vi "UART Benchmark.vi"() -> ()   [LabVIEW 2011]
uses:
  Private/Device/Device.lvlib
  Private/Type Defs/Interface.ctl
  LVH-LINX.lvlib
  <vilib>/ptbypt/NI_PtbyPt.lvlib
panel:
  in  "Data":string
  out "Device Name":string
  in  "Stop Button":bool
  out "Loop Rate":dbl(graph)
  out "Loop Time (ms)":i32
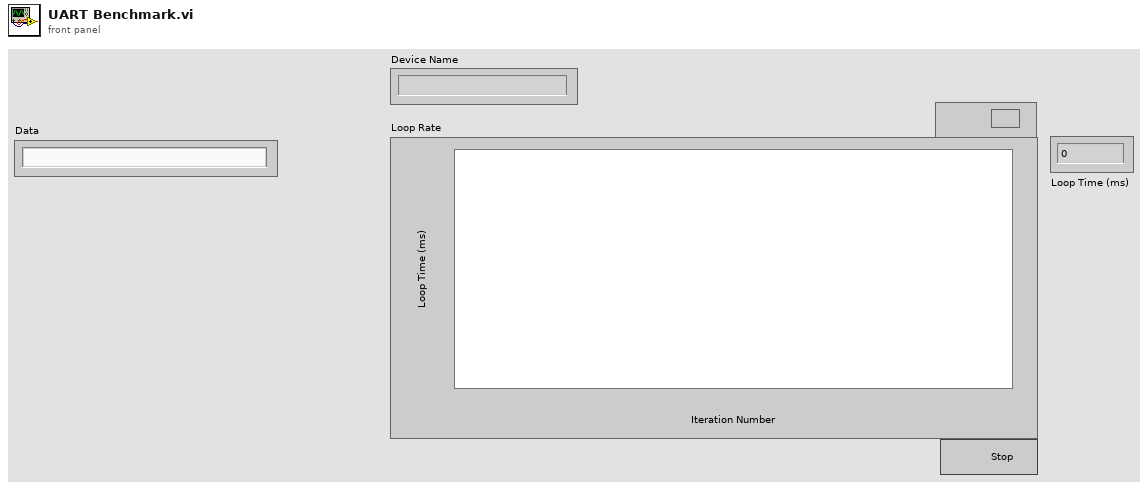
[diagram p1: front panel]
types:
  T1 = typedef "LVH-LINX.lvlib/Interface.ctl" = enum16{"Serial", "TCP"}
  T2 = typedef "LVH-LINX.lvlib/Device.lvlib/LINX Device Config.ctl" = cluster{"Interface":T1, "COM Port":refnum<visa-resource-name>, "TCP Configuration":T3, "Device Family":u8, "Device ID":u8, "Device Name":string, "TCP Ref":refnum<k5>, "Channels":T4}
  T3 = typedef "LVH-LINX.lvlib/Device.lvlib/TCP Config.ctl" = cluster{"IP Address":string, "Port":u16}
  T4 = typedef "LVH-LINX.lvlib/Channels.ctl" = cluster{"DI Channels":u8[], "DO Channels":u8[], "AI":u8[], "AO":u8[], "PWM":u8[], "QE":u8[], "UART":u8[], "I2C 2":u8[], "SPI":u8[], "CAN":u8[], "AI Ref (V)":dbl, "AO Resolution (Bits)":u8, "AO Ref (V)":dbl}
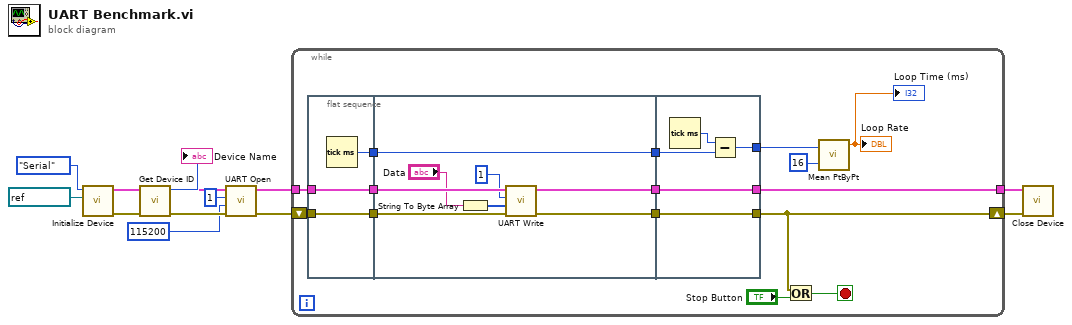
[diagram p0: block diagram]
diagram:
  n1 = call "Initialize Device.vi"("COM Port"=refnum<visa-resource-name> "COM5", "Interface"=Interface."Serial") -> ("Error Out"=w9:errorcluster, "LINX Device Config"=w10:T2)  [unwired: 8 in]
  n2 = call "Get Device ID.vi"("Error In"=w9, "LINX Device Config"=w10) -> ("Error Out"=w7:errorcluster, "Device Family"=→"Device Name":u8, "LINX Device Config"=w6:T2)  [unwired: 6 in, 1 out]
  n3 = call "UART Open.vi"("Error In"=w7, "Baud Rate (9600)"=u32 115200, "UART Channel"=u8 1, "LINX Device Config"=w6) -> ("Error Out"=w3:errorcluster, "LINX Device Config"=w2:T2)  [unwired: 6 in]
  n4 = while {
    shift-right: [w14] -> w11
    shift-left: w3 -> [w21]
    tunnel: w2 -> [w17]
    tunnel: [w16] -> w1
    stop <- w28 stop-if-true
    n5 = flat-sequence {
      tunnel: [w31] -> w26
      tunnel: w21 -> [w30]
      tunnel: [w30] -> w20
      tunnel: [w29] -> w18
      tunnel: w17 -> [w29]
      tunnel: w26 -> [w39]
      tunnel: [w39] -> w25
      tunnel: w20 -> [w38]
      tunnel: [w37] -> w19
      tunnel: w18 -> [w36]
      tunnel: [w35] -> w15
      tunnel: w25 -> [w43]
      tunnel: [w42] -> w24
      tunnel: [w41] -> w14
      tunnel: w19 -> [w41]
      tunnel: [w40] -> w16
      tunnel: w15 -> [w40]
      frame #0 {
        n6 = Tick Count (ms)() -> (millisecond timer value=w31:u32)
      }
      frame #1 {
        n7 = String To Byte Array(string="Data") -> (unsigned byte array=w33:u8[])
        n8 = call "UART Write.vi"("Error In"=w38, "Data"=w33, "UART Channel"=u8 1, "LINX Device Config"=w36) -> ("Error Out"=w37:errorcluster, "LINX Device Config"=w35:T2)  [unwired: 6 in]
      }
      frame #2 {
        n9 = Tick Count (ms)() -> (millisecond timer value=w44:u32)
        n10 = Subtract(x=w44, y=w43) -> (x-y=w42:u32)
      }
    }
    n11 = Or(x=w14, y="Stop Button") -> (x .or. y?=w28:bool)
    n12 = call <vilib>:"Mean PtByPt.vi"("x"=w24, "sample length"=16) -> ("mean"=→"Loop Rate" →"Loop Time (ms)":dbl)  [unwired: 2 in, 1 out]
  }
  n13 = call "Close Device.vi"("Error In"=w11, "LINX Device Config"=w1) -> ()  [unwired: 8 in, 2 out]
